vi "Close Context.vi"(8 "error in (no error)":errorcluster, 11 "App":refnum<vi>) -> (0 "error out":errorcluster)   [LabVIEW 2020, in "LV-Protoc.lvlib"]
uses:
  LV-Protoc.lvlib
panel:
  out "RefCount":i32
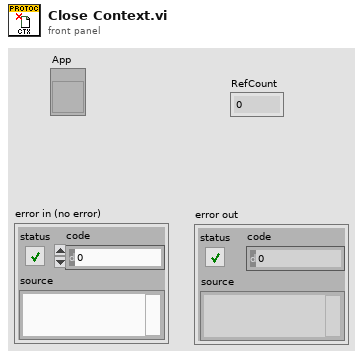
[diagram p1: front panel]
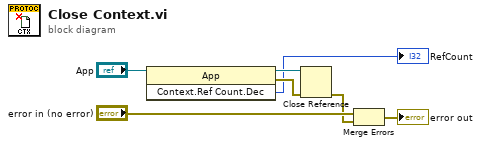
[diagram p0: block diagram]
diagram:
  n1 = invoke class="App" method="Context.Ref Count.Dec"(reference="App") -> (reference out=w6:refnum<vi>, error out=w7:errorcluster, "Context.Ref Count.Dec"=→"RefCount":i32)  [unwired: 2 in]
  n2 = Close Reference(reference=w6, error in (no error)=w7) -> (error out=w2:errorcluster)
  n3 = Merge Errors("error in (no error)", w2) -> (→"error out":errorcluster)
